vi "Write Variance.vi"(8 "error in (no error)":errorcluster, 10 "Variance":dbl, 11 "Standard Averager in":refnum<class "Standard Averager.lvclass">) -> (0 "error out":errorcluster, 3 "Standard Averager out":refnum<class "Standard Averager.lvclass">)   [LabVIEW 2018, in "Standard Averager.lvclass"]
uses:
  Standard Averager.lvclass
  Standard Averager.lvclass/Standard Averager.ctl
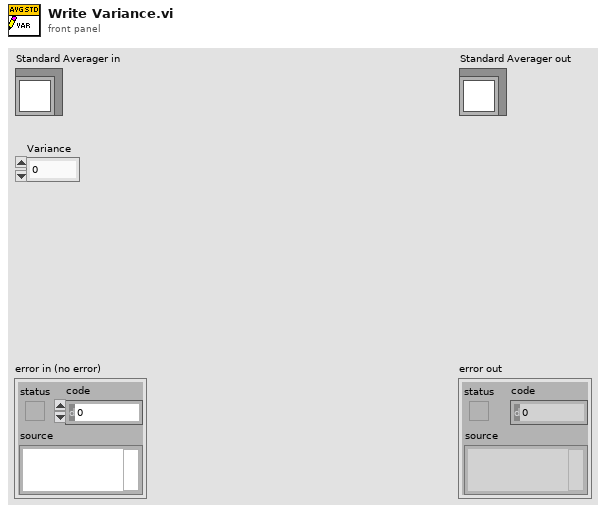
[diagram p1: front panel]
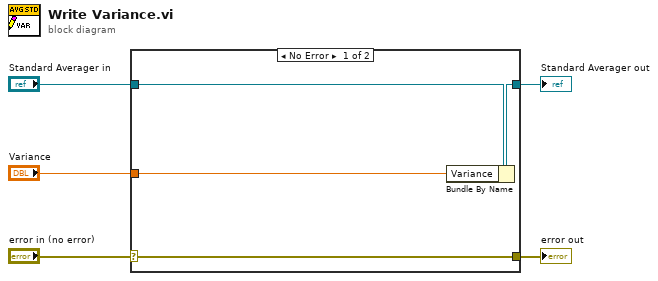
[diagram p0: block diagram]
diagram:
  n1 = case shown="No Error" "error in (no error)" {
    selector: "error in (no error)" -> [w9 w10]
    tunnel: [w9 w10] -> w4
    tunnel: [w7 w11] -> w2
    tunnel: "Standard Averager in" -> [w8 w11]
    tunnel: "Variance" -> [w6 _]
    frame No Error {
      n2 = Bundle By Name(cluster=w8, "Variance"=w6) -> (w7:refnum<class "Standard Averager.lvclass">)
    }
    frame Error {
    }
  }
  "error out" <- w4
  "Standard Averager out" <- w2
